vi "Open File.vi"(7 "Append If Existing File":bool, 8 "error in (no error)":errorcluster, 10 "Method (Read)":enum16{"Write", "Read"}(ring)=enum."Read", 11 "Log Path":path) -> (0 "error out":errorcluster, 3 "BLF File":refnum<class "Read Write BLF.lvclass">)   [LabVIEW 2015, in "Read Write BLF.lvclass"]
doc: "This VI will open a <B>BLF File</B>. This function allows for Reading, or Writing but not both in one session. Enter the <B>Log Path</B>, along with the <B>Method</B> which defaults to Read. This function is writing a file it will default to creating a new file, even if the file already exists. Use the <B>Append If Existing File</B> setting it to True to cause it to read the contents of the file before deleting it and then write those contents. This will only read and only write CAN Frames so if other data objects are stored in the file they will be lost.\n\n-------------\nBrian Hoover (Hooovahh)"
uses:
  Read Write BLF.lvclass
  Read Write BLF.lvclass/Read Write BLF.ctl
  Write CAN Frame.vi
  Set Measurement Start Time.vi
  <vilib>/Utility/file.llb/Application Directory.vi
  <vilib>/Utility/error.llb/Error Cluster From Error Code.vi
  <vilib>/ErrorRing/Error Ring.xnode
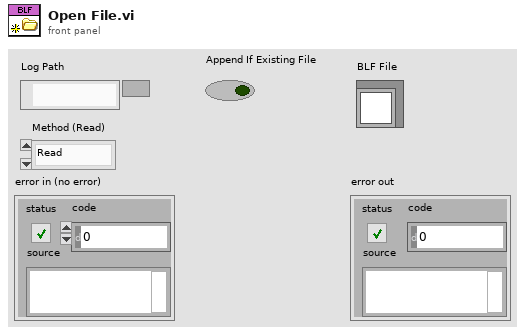
[diagram p1: front panel]
types:
  T1 = typedef "Read Write BLF.lvclass/Cluster - Application Information.ctl" = cluster{"Application ID":T2, "Major":u8, "Minor":u8, "Build":u8}
  T2 = typedef "Read Write BLF.lvclass/Enum - Application ID.ctl" = enum8{"UNKNOWN", "CANALYZER", "CANOE", "CANSTRESS", "CANLOG", "CANAPE", "CANCASEXLLOG"}
  T3 = typedef "Read Write BLF.lvclass/Cluster - CAN Frame.ctl" = cluster{"timestamp":timestamp, "payload":u8[], "identifier":u32, "extended?":bool, "echo?":bool, "type":T4}
  T4 = typedef "Read Write BLF.lvclass/Enum - CAN Data Type.ctl" = u8
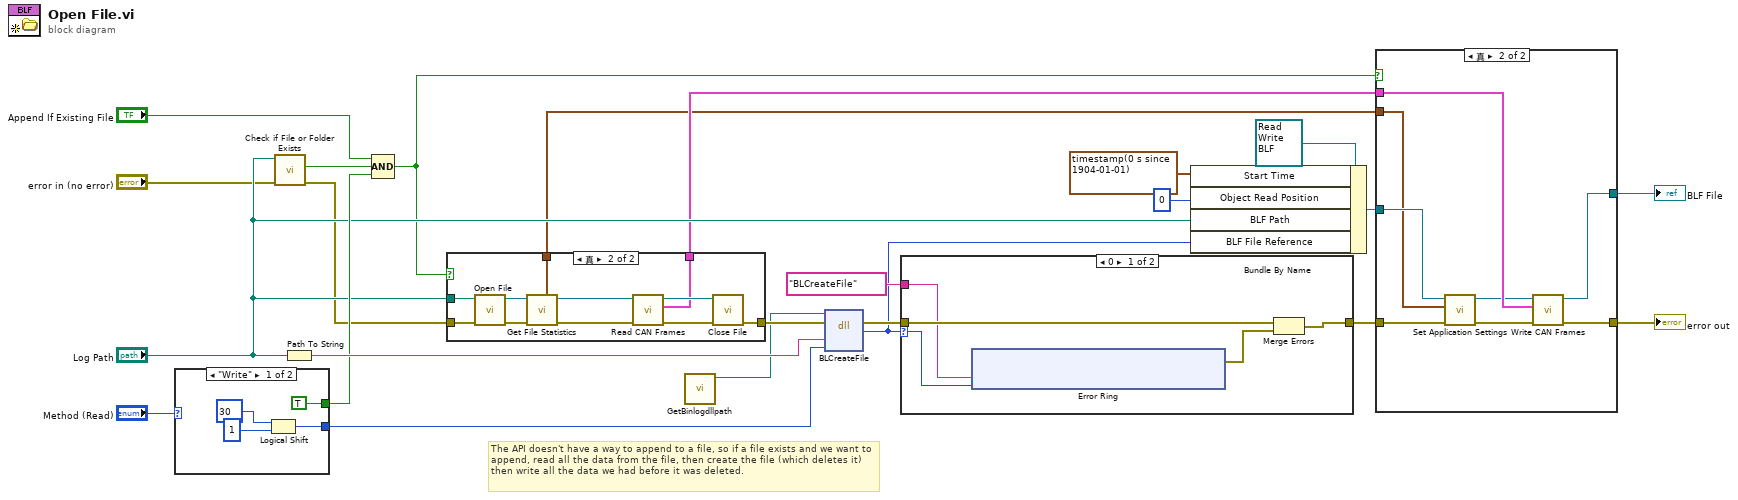
[diagram p0: block diagram]
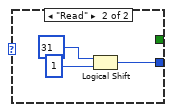
[diagram p5: hidden frame]
diagram:
  # "The API doesn't have a way to append to a file, so if a file exists and we want to append, read all the data from the file, then create the file (which deletes it) then write all the data we had before it was deleted."
  n1 = case shown="\"Write\"" "Method (Read)" {
    tunnel: [w26 w29] -> w22
    tunnel: [TRUE _] -> w13
    frame "Write" {
      n2 = Logical Shift(y=i16 30, x=u32 1) -> (x << y=w26:u32)
    }
    frame "Read" {
      n3 = Logical Shift(y=i16 31, x=u32 1) -> (x << y=w29:u32)
    }
  }
  n4 = call <vilib>:"Check if File or Folder Exists.vi"("error in (no error)"="error in (no error)", "path"="Log Path") -> ("error out"=w3:errorcluster, "file or folder exists?"=w15:bool)  [unwired: 7 in, 1 out]
  n5 = Path To String(path="Log Path") -> (string=w24:string)
  n6 = Compound Arithmetic op=AND("Append If Existing File", w15, w13) -> (w5:bool)
  n7 = case shown="真" w5 {
    tunnel: w3 -> [w32 w43]
    tunnel: [w32 w39] -> w12
    tunnel: "Log Path" -> [_ w41]
    tunnel: [_ w37] -> w7
    tunnel: [_ w33] -> w2
    frame False {
    }
    frame True {
      n8 = call "Open File.vi"("error in (no error)"=w43, "Log Path"=w41) -> ("error out"=w42:errorcluster, "BLF File"=w35:refnum<class "Read Write BLF.lvclass">)  [unwired: 8 in]
      n9 = call "Get File Statistics.vi"("error in (no error)"=w42, "Read Write BLF in"=w35) -> ("error out"=w36:errorcluster, "Read Write BLF out"=w34:refnum<class "Read Write BLF.lvclass">, "Application Information"=w33:T1)  [unwired: 3 in, 4 out]
      n10 = call "Read CAN Frames.vi"("error in (no error)"=w36, "BLF File In"=w34) -> ("error out"=w40:errorcluster, "CAN Frames"=w37:T3[], "BLF File Out"=w38:refnum<class "Read Write BLF.lvclass">)  [unwired: 6 in, 1 out]
      n11 = call "Close File.vi"("error in (no error)"=w40, "BLF File"=w38) -> ("error out"=w39:errorcluster)  [unwired: 8 in, 1 out]
    }
  }
  n12 = call "GetBinlogdllpath.vi"() -> ("dup path"=w1:path)  [unwired: 11 in]
  n13 = dll-call lib="PTH2Xabs E自开发软件X-CAN项目 X-CAN离线分析平台 V2.2.8.0BLF\nbinlog.dll" fn="BLCreateFile"(path in=w1, error in=w12, "lpFileName"=w24, "dwDesiredAccess"=w22) -> (error out=w21:errorcluster, "return type"=w18:u32)  [unwired: 3 in, 1 out]
  n14 = case shown="0" w18 {
    selector: w18 -> [w45 _]
    tunnel: w21 -> [w48 w57]
    tunnel: [w47 w57] -> w10
    tunnel: "BLCreateFile" -> [w44 _]
    frame 0 {
      n15 = xnode "Error Ring"("参数 0"=w44, "参数 1"=w45) -> ("错误输出"=w46:errorcluster)
      n16 = Merge Errors(w48, w46) -> (w47:errorcluster)
    }
    frame Default {
    }
  }
  n17 = Bundle By Name(cluster=refnum<class "Read Write BLF.lvclass"> refnum ("BLF File"), "Start Time"=timestamp(0 s since 1904-01-01), "Object Read Position"=u32 0, "BLF Path"="Log Path", "BLF File Reference"=w18) -> (w9:refnum<class "Read Write BLF.lvclass">)
  n18 = case shown="真" w5 {
    tunnel: w10 -> [w58 w67]
    tunnel: w9 -> [w59 w62]
    tunnel: [w58 w66] -> w8
    tunnel: w7 -> [_ w65]
    tunnel: [w59 w64] -> w6
    tunnel: w2 -> [_ w60]
    frame False {
    }
    frame True {
      n19 = call "Set Application Settings.vi"("error in (no error)"=w67, "Application Information"=w60, "BLF File In"=w62) -> ("error out"=w63:errorcluster, "BLF File Out"=w61:refnum<class "Read Write BLF.lvclass">)  [unwired: 7 in]
      n20 = call "Write CAN Frames.vi"("error in (no error)"=w63, "Frames"=w65, "Read Write BLF in"=w61) -> ("error out"=w66:errorcluster, "Read Write BLF out"=w64:refnum<class "Read Write BLF.lvclass">)  [unwired: 7 in]
    }
  }
  "error out" <- w8
  "BLF File" <- w6
